vi "LEAPread.vi"(8 "error in (no error)":errorcluster, 11 "Controller Refnum In":refnum<k24>) -> (0 "error out":errorcluster, 1 "IsConnected":bool, 2 "Frame":T1, 3 "Controller Refnum Out":refnum<k24>, 5 "Hand count":i32)   [LabVIEW 2017, in "LeapMotion.lvlib"]
uses:
  LeapMotion.lvlib
  C:/Users/Sara/Documents/GitHub/LEAP-sign-language/LEAP-sign-language/LeapMotion/Dynamic Libraries/LeapCSharp.NET4.5.dll
  Dynamic Libraries/LeapCSharp.NET4.5.dll
  TypeDefs/LEAPframe.ctl
  TypeDefs/LEAPhand.ctl
  TypeDefs/LEAParm.ctl
  TypeDefs/LEAPvector.ctl
  TypeDefs/LEAPfinger.ctl
  TypeDefs/LEAPbone.ctl
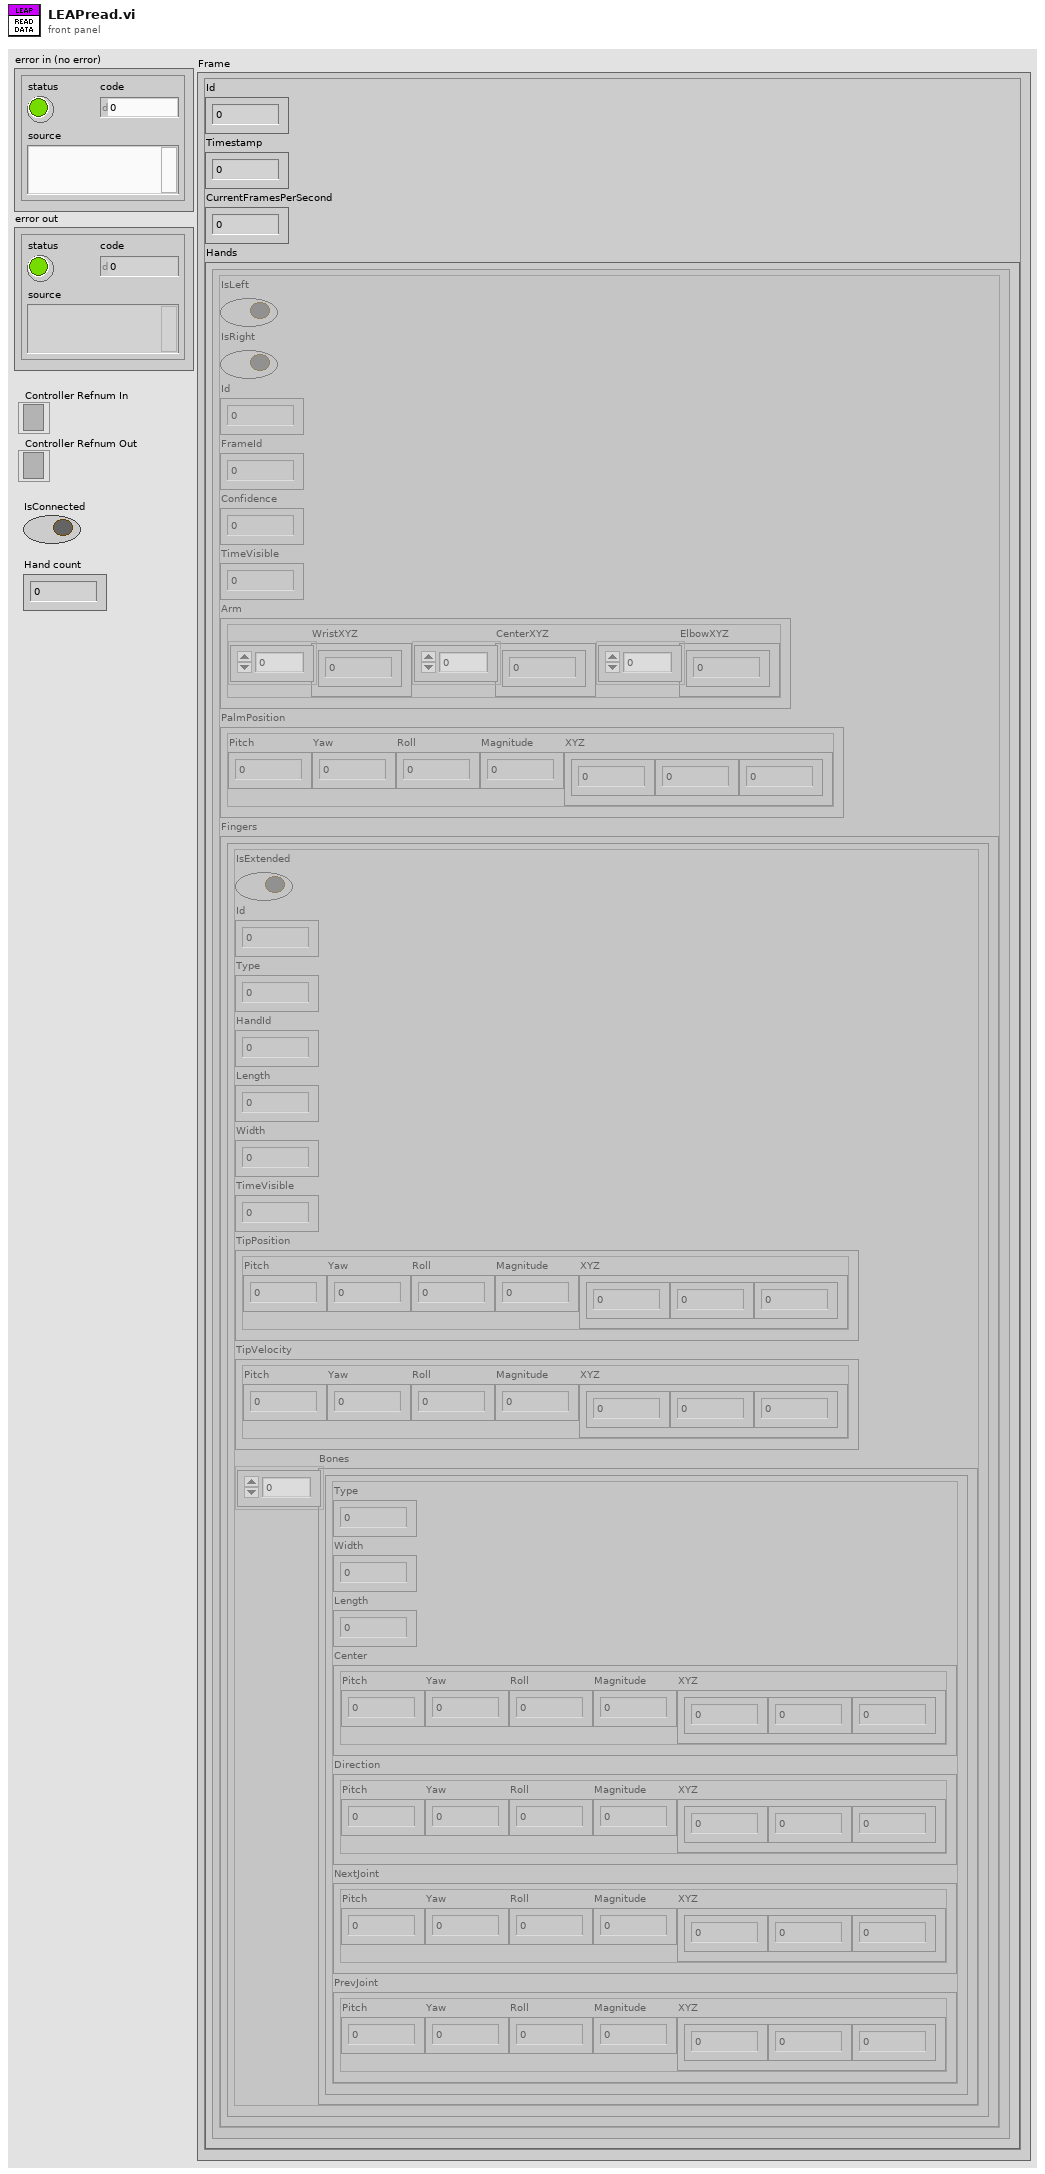
[diagram p1: front panel]
types:
  T1 = typedef "LeapMotion.lvlib/LEAPframe.ctl" = cluster{"Id":i64, "Timestamp":i64, "CurrentFramesPerSecond":sgl, "Hands":T2[]}
  T2 = typedef "LeapMotion.lvlib/LEAPhand.ctl" = cluster{"IsLeft":bool, "IsRight":bool, "Id":i32, "FrameId":i64, "Confidence":sgl, "TimeVisible":sgl, "Arm":T3, "PalmPosition":T4, "Fingers":T5[]}
  T3 = typedef "LeapMotion.lvlib/LEAParm.ctl" = cluster{"WristXYZ":sgl[], "CenterXYZ":sgl[], "ElbowXYZ":sgl[]}
  T4 = typedef "LeapMotion.lvlib/LEAPvector.ctl" = cluster{"Pitch":sgl, "Yaw":sgl, "Roll":sgl, "Magnitude":sgl, "XYZ":sgl[]}
  T5 = typedef "LeapMotion.lvlib/LEAPfinger.ctl" = cluster{"IsExtended":bool, "Id":i32, "Type":i32, "HandId":i32, "Length":sgl, "Width":sgl, "TimeVisible":sgl, "TipPosition":T4, "TipVelocity":T4, "Bones":T6[]}
  T6 = typedef "LeapMotion.lvlib/LEAPbone.ctl" = cluster{"Type":i32, "Width":sgl, "Length":sgl, "Center":T4, "Direction":T4, "NextJoint":T4, "PrevJoint":T4}
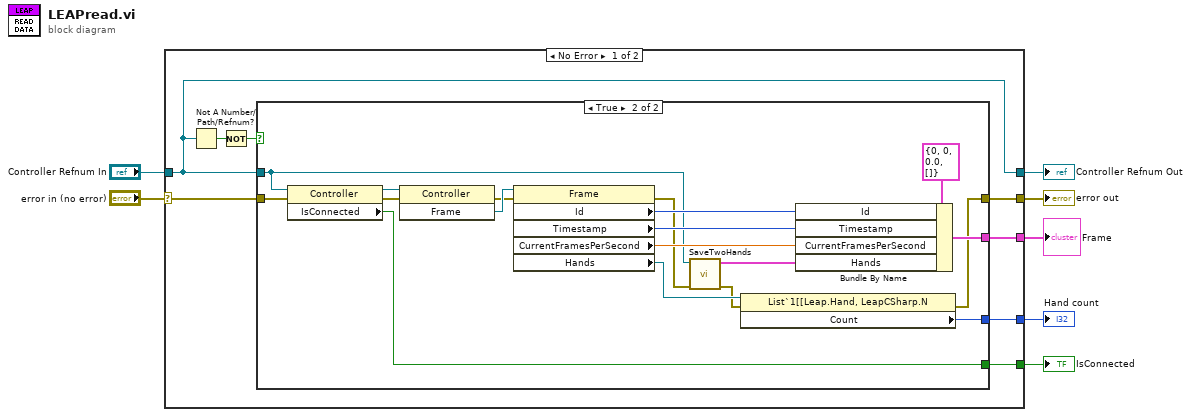
[diagram p0: block diagram]
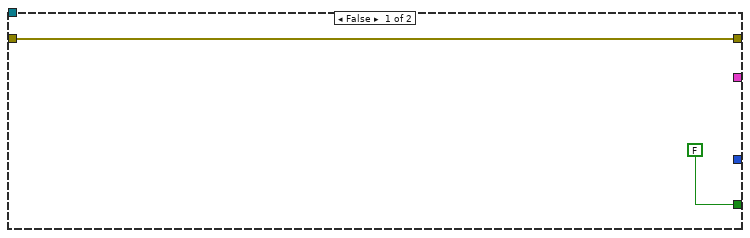
[diagram p2: hidden frame]
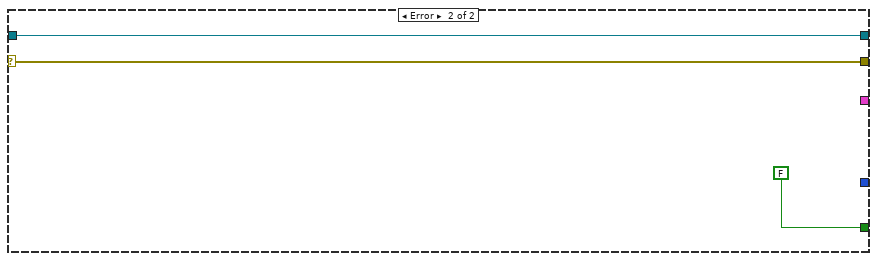
[diagram p3: hidden frame]
diagram:
  n1 = case shown="No Error" "error in (no error)" {
    selector: "error in (no error)" -> [w13 w37]
    tunnel: "Controller Refnum In" -> [w9 w36]
    tunnel: [w9 w36] -> w5
    tunnel: [w12 FALSE ("IsConnected")] -> w6
    tunnel: [w11 w37] -> w7
    tunnel: [w10 _] -> w2
    tunnel: [w8 _] -> w1
    frame No Error {
      n2 = Not A Number/Path/Refnum?(number/path/refnum=w9) -> (NaN/Path/Refnum?=w15:bool)
      n3 = Not(x=w15) -> (.not. x?=w14:bool)
      n4 = case shown="True" w14 {
        tunnel: w13 -> [w16 w35]
        tunnel: w9 -> [_ w23]
        tunnel: [FALSE ("IsConnected") w32] -> w12
        tunnel: [w16 w18] -> w11
        tunnel: [_ w25] -> w10
        tunnel: [_ w20] -> w8
        frame False {
        }
        frame True {
          n5 = property class="Controller"(reference=w23, error in=w35) -> (reference out=w33:refnum<k24>, error out=w34:errorcluster, "IsConnected"=w32:bool)
          n6 = invoke class="Controller" method="Frame"(reference=w33, error in=w34) -> (error out=w30:errorcluster, "Frame"=w31:refnum<k24>)  [unwired: 1 in, 1 out]
          n7 = property class="Frame"(reference=w31, error in=w30) -> (error out=w22:errorcluster, "Id"=w28:i64, "Timestamp"=w27:i64, "CurrentFramesPerSecond"=w26:sgl, "Hands"=w21:refnum<k24>)  [unwired: 1 out]
          n8 = call "SaveTwoHands.vi"("error in (no error)"=w22, "Leap.Controller"=w23) -> ("error out"=w19:errorcluster, "Hand array"=w24:T2[])  [unwired: 8 in]
          n9 = property class="List`1[[Leap.Hand, LeapCSharp.N"(reference=w21, error in=w19) -> (error out=w18:errorcluster, "Count"=w20:i32)  [unwired: 1 out]
          n10 = Bundle By Name(cluster=T1 {"Id"=0, "Timestamp"=0, "CurrentFramesPerSecond"=0.0, "Hands"=[]} ("Frame"), "Id"=w28, "Timestamp"=w27, "CurrentFramesPerSecond"=w26, "Hands"=w24) -> (w25:T1)
        }
      }
    }
    frame Error {
    }
  }
  "error out" <- w7
  "IsConnected" <- w6
  "Controller Refnum Out" <- w5
  "Frame" <- w2
  "Hand count" <- w1
